vi "2022.12.5-边缘检测-斑点.vi"() -> ()   [LabVIEW 2018]
uses:
  <vilib>/vision/NI_Vision_Development_Module.lvlib
panel:
  in  "Settings":T1={"Objects"=0, "Threshold"=128, "Reject Border"=FALSE, "Fill Holes"=FALSE, "Min Object Size"=FALSE, "Min Size"=3, "Max Object Size"=FALSE, "Max Size"=100, "Show Search Area"=FALSE, "Show Center"=TRUE, "Show Bounding Box"=TRUE} {"Objects" items=["Bright Objects", "Dark Objects"]; "Threshold" min=1 max=999999999 step=1; "Max Size" min=1 max=999999999 step=1; "Min Size" min=1 max=999999999 step=1}
  out "Objects":T2(array[cluster]) {"Aspect Ratio" format="%.2f"; "Orientation" format="%.2f"; "Area" format="%.2f"; "Object Center"."Y" format="%.2f"; "Object Center"."X" format="%.2f"}
  in  "停止":bool
  out "Image":T3(plugin-control)
  out "Coordinate System (duplicate)":T4 {"Measurement System"."Axis Reference" items=["Direct", "Indirect"]; "Measurement System"."Angle (deg)" format="%.2f"; "Measurement System"."Origin"."Y" format="%.2f"; "Measurement System"."Origin"."X" format="%.2f"; "Reference System"."Axis Reference" items=["Direct", "Indirect"]; "Reference System"."Angle (deg)" format="%.2f"; "Reference System"."Origin"."Y" format="%.2f"; "Reference System"."Origin"."X" format="%.2f"}
  in  "File Path":path
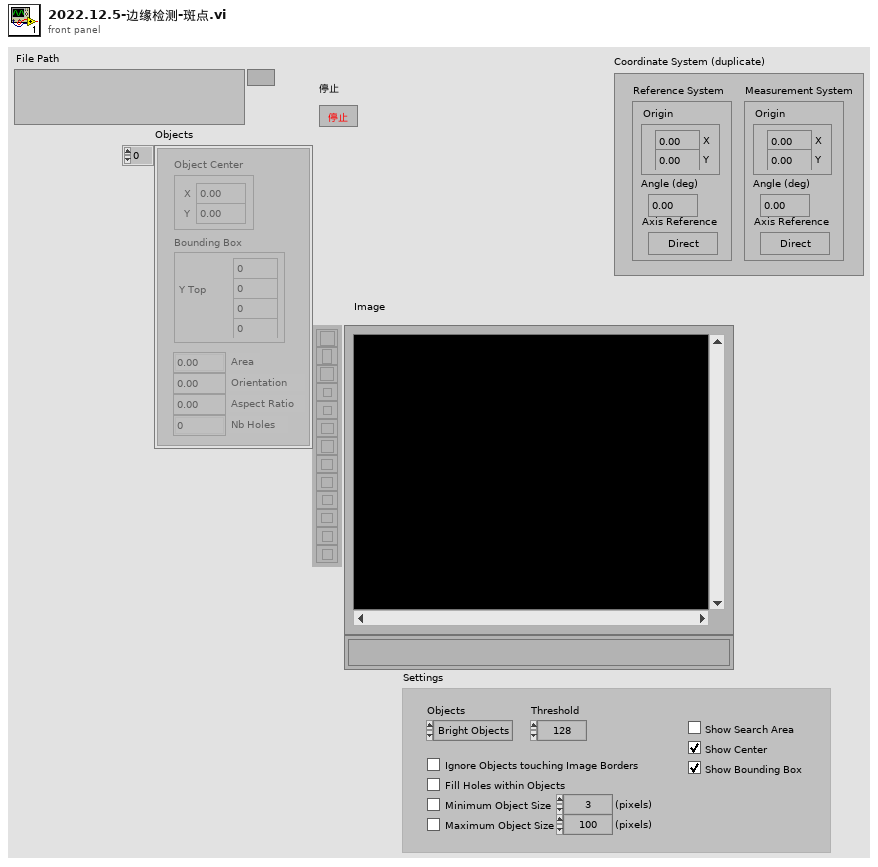
[diagram p1: front panel]
types:
  T1 = cluster{"Objects":u16, "Threshold":i32, "Reject Border":bool, "Fill Holes":bool, "Min Object Size":bool, "Min Size":i32, "Max Object Size":bool, "Max Size":i32, "Show Search Area":bool, "Show Center":bool, "Show Bounding Box":bool}
  T2 = cluster{"Object Center":cluster{"X":sgl, "Y":sgl}, "Bounding Box":cluster{"X Left":i32, "Y Top":i32, "X Right":i32, "Y Bottom":i32}, "Area":sgl, "Orientation":sgl, "Aspect Ratio":sgl, "Nb Holes":i32}[]
  T3 = typedef "IMAQ Image.ctl" = refnum<image>
  T4 = typedef "IMAQ Coordinate System" = cluster{"Reference System":cluster{"Origin":cluster{"X":sgl, "Y":sgl}, "Angle (deg)":sgl, "Axis Reference":u32}, "Measurement System":cluster{"Origin":cluster{"X":sgl, "Y":sgl}, "Angle (deg)":sgl, "Axis Reference":u32}}
  T5 = typedef "Image Type" = u32
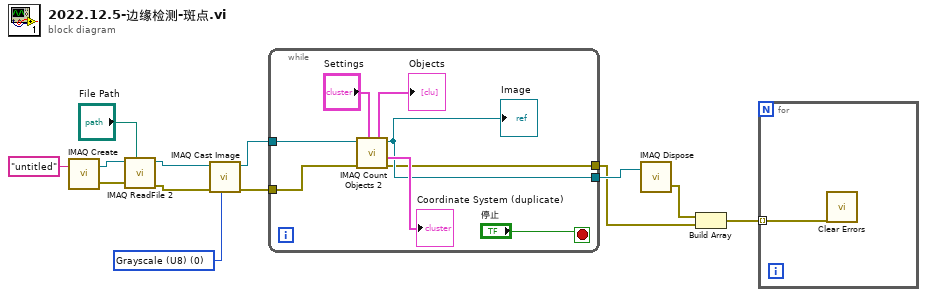
[diagram p0: block diagram]
diagram:
  w7 = T5 0 items=["Grayscale (U8)", "Grayscale (I16)", "Grayscale (SGL)", "Complex (CSG)", "RGB (U32)", "HSL (U32)", "RGB (U64)", "Grayscale (U16)"] ("Image Type")
  n1 = call "IMAQ Create"("Image Name"="untitled") -> ("New Image"=w13:T3, "error out"=w12:errorcluster)  [unwired: 4 in]
  n2 = call "IMAQ ReadFile 2"("File Path"="File Path", "error in (no error)"=w12, "Image"=w13) -> ("error out"=w8:errorcluster, "Image Out"=w9:T3)  [unwired: 4 in, 3 out]
  n3 = call "IMAQ Cast Image"("Image Type"=w7, "error in (no error)"=w8, "Image Src"=w9) -> ("error out"=w5:errorcluster, "Image Dst Out"=w6:T3)  [unwired: 7 in]
  n4 = while {
    tunnel: w6 -> [w21]
    tunnel: w5 -> [w20]
    tunnel: [w18] -> w4
    tunnel: [w16] -> w1
    stop <- "停止" stop-if-true
    n5 = call "IMAQ Count Objects 2"("Settings"="Settings", "error in (no error)"=w20, "Image"=w21) -> ("error out"=w16:errorcluster, "Coordinate System (duplicate)"=→"Coordinate System (duplicate)":T4, "Image Out"=w18:T3, "Objects"=→"Objects":T2)  [unwired: 4 in, 1 out]
    "Image" <- w18
  }
  n6 = call "IMAQ Dispose"("Image"=w4) -> ("error out"=w3:errorcluster)  [unwired: 5 in]
  n7 = Build Array(w3, w1) -> (w2:errorcluster[])
  n8 = for {
    tunnel: w2 -> [w22] mode=indexing
    n9 = call <vilib>:"Clear Errors.vi"("error in (no error)"=w22) -> ()  [unwired: 5 in, 2 out]
  }
